vi "Run VI Test Alyssa.vi"(11 "Array":string[](array[string])) -> (2 "String":string, 3 "Numeric":i32)   [LabVIEW 2018]
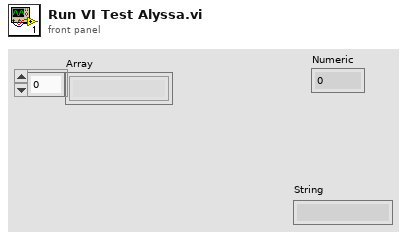
[diagram p1: front panel]
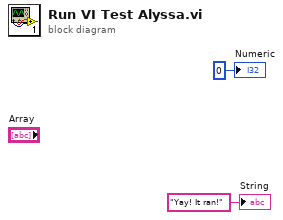
[diagram p0: block diagram]
diagram:
  "String" <- "Yay! It ran!" ("String")
  "Numeric" <- 0 ("Numeric")
